vi "Blink Test.vi"() -> ()   [LabVIEW 2021]
panel:
  out "Clock Output":bool
  out "Elapsed mS":u32
  out "SampleDelay":u32
  in  "Flip":bool
  in  "Stop Button":bool
  in  "Blink Two":bool
  in  "Blink One":bool
  out "Blink Two":bool
  out "Blink One":bool
  in  "Delay Two":u32
  in  "Delay One":u32
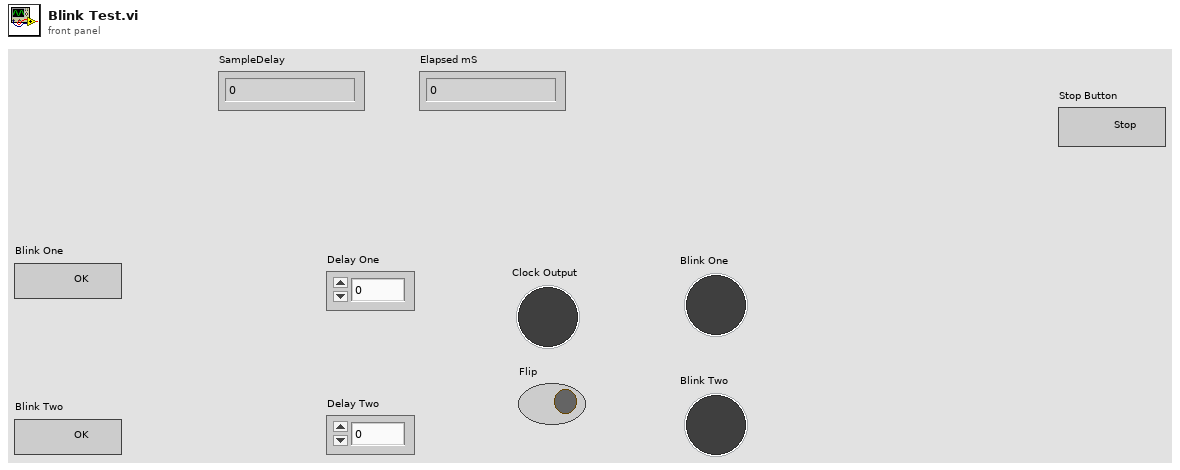
[diagram p1: front panel]
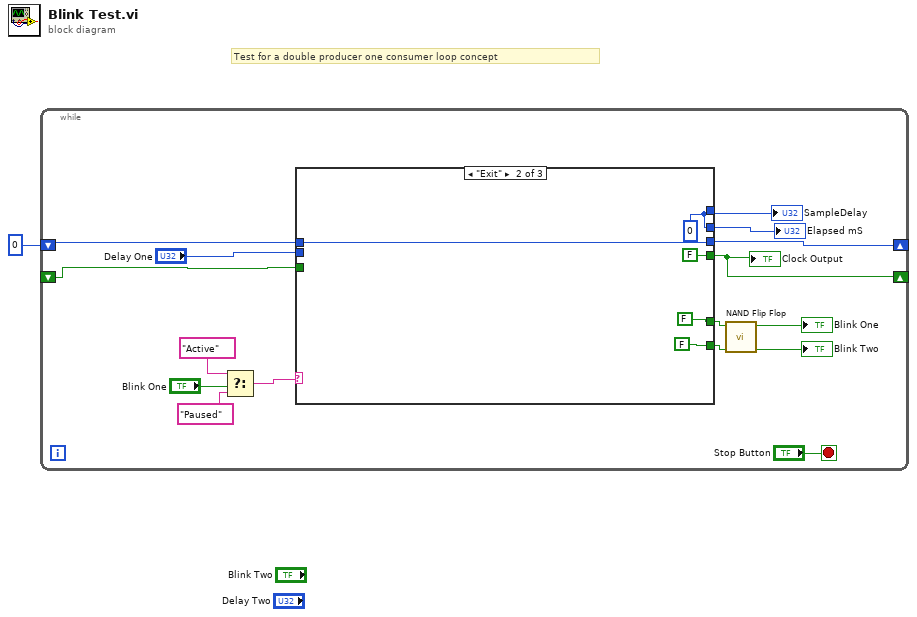
[diagram p0: block diagram]
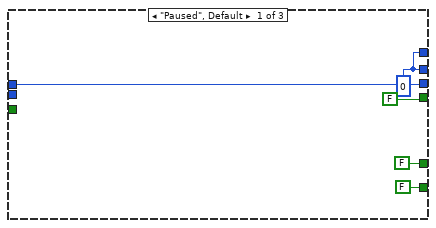
[diagram p2: hidden frame]
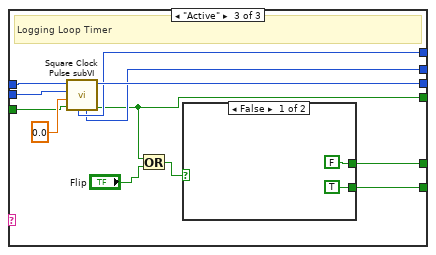
[diagram p3: hidden frame]
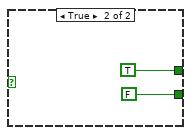
[diagram p4: hidden frame]
diagram:
  # "Test for a double producer one consumer loop concept"
  n1 = while {
    shift-right: [w16] -> _
    shift-left: u32 0 ("Last Event mS") -> [w17]
    shift-right: [w2] -> _
    shift-left: _ -> [w3]
    stop <- "Stop Button" stop-if-true
    n2 = Select(t="Active", s="Blink One", f="Paused") -> (s? t:f=w14:string)
    n3 = case shown="\"Exit\"" w14 {
      tunnel: [w22 w27 w38] -> w16
      tunnel: w17 -> [w22 w27 w37]
      tunnel: [FALSE FALSE ("Blink One") w36] -> w8
      tunnel: [FALSE ("Reset") FALSE ("Reset") w35] -> w7
      tunnel: "Delay One" -> [_ _ w29]
      tunnel: [w19 w24 w32] -> w5
      tunnel: [w19 w24 w31] -> w4
      tunnel: [FALSE ("Clock Output") FALSE ("Clock Output") w28] -> w2
      tunnel: w3 -> [_ _ w30]
      frame "Paused", Default {
        w19 = u32 0 ("Elapsed mS")
      }
      frame "Exit" {
        w24 = u32 0 ("SampleDelay")
      }
      frame "Active" {
        # "Logging Loop Timer"
        n4 = call "Square Clock Pulse subVI.vi"("Last Bool State"=w30, "Sample Rate (Hz)"=0.0, "SampleDelay(in)"=w29, "Last Event mS"=w37) -> ("Clock Output"=w28:bool, "Last Event mS"=w38:u32, "Elapsed mS"=w31:u32, "SampleDelay"=w32:u32)  [unwired: 4 in]
        n5 = Or(x=w28, y="Flip") -> (x .or. y?=w34:bool)
        n6 = case shown="False" w34 {
          tunnel: [FALSE ("Blink One") TRUE ("Blink One")] -> w36
          tunnel: [TRUE ("Reset") FALSE ("Reset")] -> w35
          frame False {
          }
          frame True {
          }
        }
      }
    }
    "SampleDelay" <- w5
    "Elapsed mS" <- w4
    "Clock Output" <- w2
    n7 = call "NAND Flip Flop.vi"("Reset"=w7, "Set"=w8) -> ("!Q"=→"Blink Two":bool, "Q"=→"Blink One":bool)  [unwired: 8 in]
  }
